vi "AutoAnneal.vi"(0 "VISA resource name":refnum<visa-resource-name>, 1 "Preheat Current":dbl format="%.3f", 5 "Ouput(On:T)":bool=TRUE, 7 "Current Mode(Immediate:F)":bool, 9 "Voltage Mode(Immediate:F)":bool, 11 "error in (no error)":errorcluster, 12 "Voltage":dbl=8.19 format="%.3f", 13 "Preheat Ramp Delay":u32=1000, 14 "Protection(None:0)":u16(ring) items=["None", "Overcurrent protection", "Overvoltage protection", "Overcurrent and overvoltage protection", "Clear overvoltage condition", "Clear overcurrent protection", "Set time delay"]) -> ()   [LabVIEW 2012]
doc: "The Application Example configures, triggers (after a user defined time delay) and stores the setting to a user defined address."
uses:
  Agilent 66XX Series.lvlib
panel:
  in  "Ramp Down Step Size":dbl=0.005 format="%.3f"
  in  "Ramp Down Delay":u32=2000
  in  "Anneal Time":dbl=5.0 format="%.3f"
  out "Anneal Current 2":dbl(graph)
  out "error out":errorcluster
  in  "Preheat Time":dbl=5.0 format="%.3f"
  in  "Overvoltage prot value":dbl=5.0 format="%.3f"
  in  "Anneal Current":dbl format="%.3f"
  in  "Anneal Step Size":dbl=0.005 format="%.3f"
  in  "Anneal Ramp Delay":u32=2000
  out "Anneal Current":dbl(graph)
  out "Preheat Current":dbl(graph)
  in  "START":bool
  in  "Preheat Step Size":dbl=0.1 format="%.3f"
  in  "Reset (F:no)":bool
  in  "ID query (T:yes)":bool=TRUE
  # "Power Supply Configurations"
  # "Preheat Settings"
  # "Amps"
  # "min"
  # "ms"
  # "Amps/Step"
  # "ms"
  # "Anneal Settings"
  # "Ramp Down Settings"
  # "Amps/Step"
  # "Yes"
  # "No"
  # "Yes"
  # "No"
  # "Trigger"
  # "Immediate"
  # "Trigger"
  # "Immediate"
  # "On"
  # "Off"
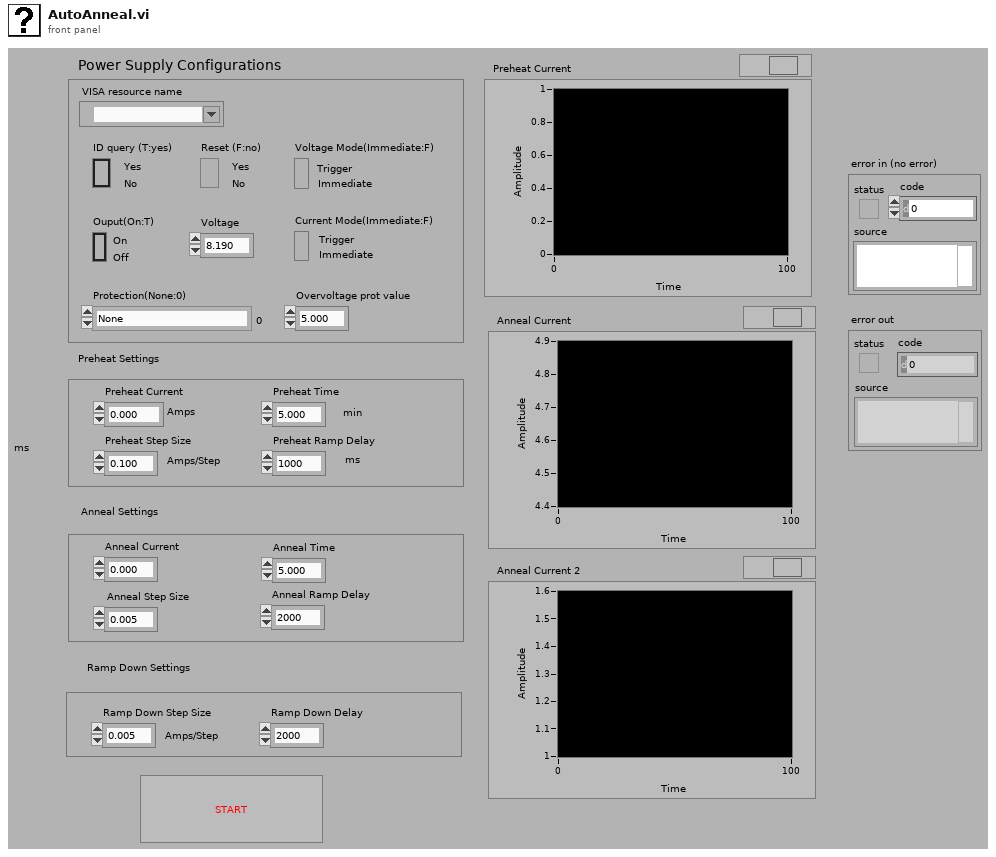
[diagram p1: front panel]
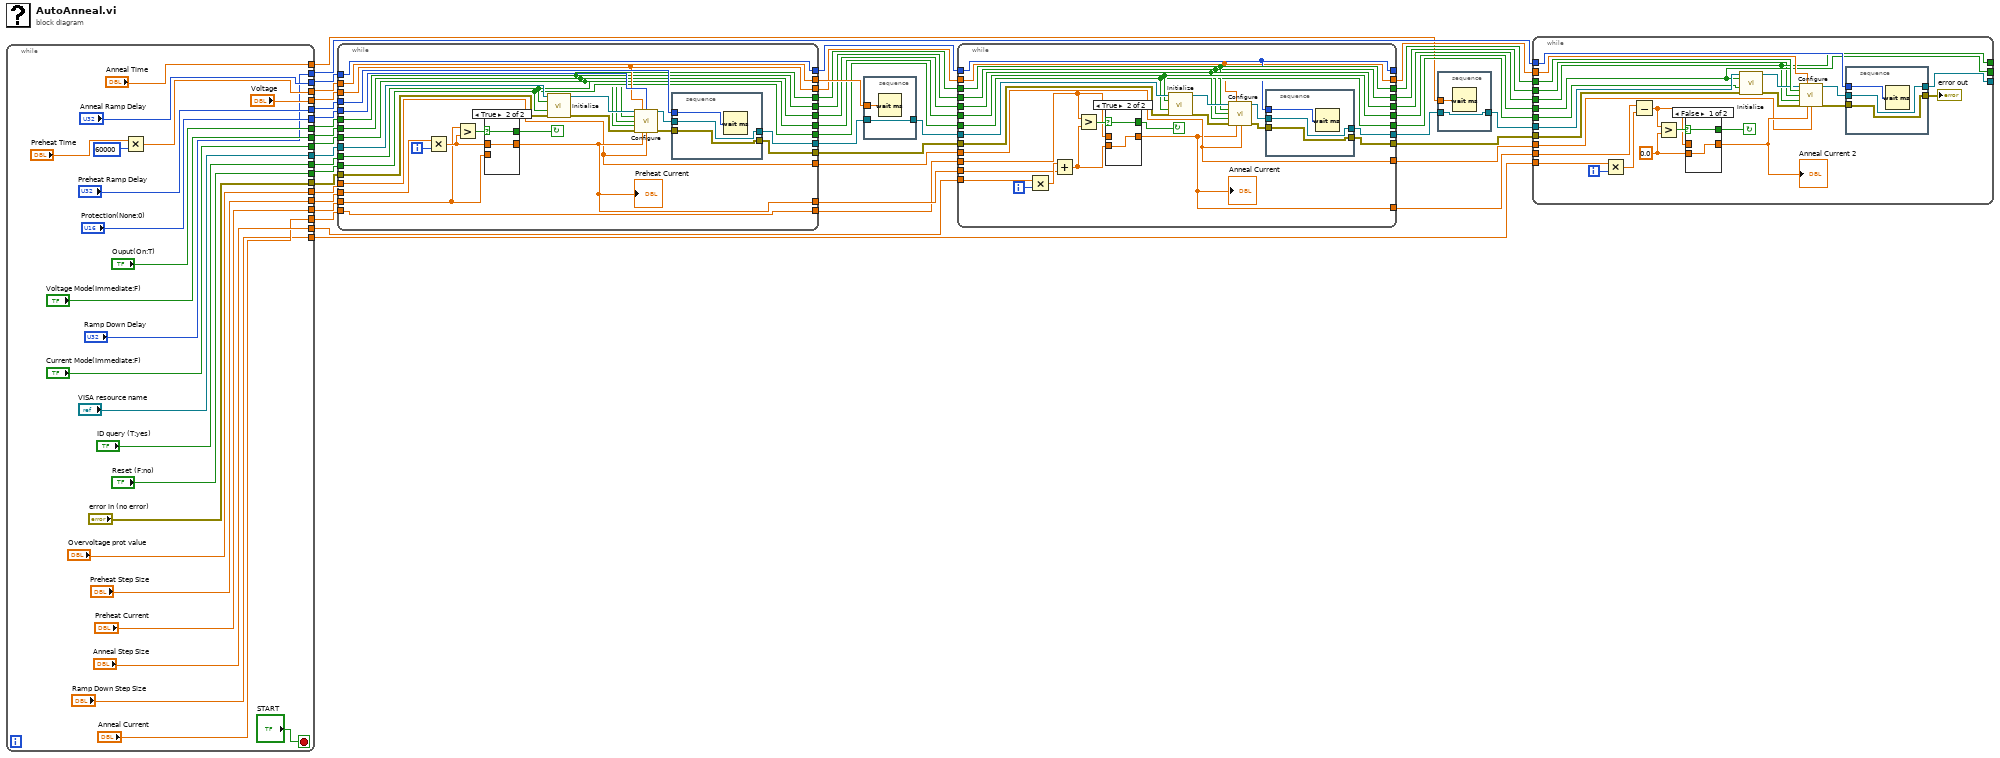
[diagram p0: block diagram]
diagram:
  n1 = while {
    tunnel: ["Current Mode(Immediate:F)"] -> w45
    tunnel: ["Voltage Mode(Immediate:F)"] -> w44
    tunnel: ["Ouput(On:T)"] -> w43
    tunnel: ["Voltage"] -> w42
    tunnel: ["Protection(None:0)"] -> w41
    tunnel: ["Preheat Current"] -> w40
    tunnel: ["Preheat Ramp Delay"] -> w39
    tunnel: ["VISA resource name"] -> w38
    tunnel: ["ID query (T:yes)"] -> w37
    tunnel: ["Reset (F:no)"] -> w36
    tunnel: ["error in (no error)"] -> w35
    tunnel: ["Preheat Step Size"] -> w34
    tunnel: [w50] -> w32
    tunnel: ["Anneal Ramp Delay"] -> w30
    tunnel: ["Anneal Step Size"] -> w24
    tunnel: ["Anneal Current"] -> w22
    tunnel: ["Overvoltage prot value"] -> w16
    tunnel: ["Ramp Down Step Size"] -> w3
    tunnel: ["Ramp Down Delay"] -> w2
    tunnel: ["Anneal Time"] -> w1
    stop <- "START" stop-if-true
    n2 = Multiply(x="Preheat Time", y=60000) -> (x*y=w50:dbl)
  }
  n3 = while {
    tunnel: w45 -> [w73]
    tunnel: w44 -> [w72]
    tunnel: w43 -> [w71]
    tunnel: w42 -> [w80]
    tunnel: w41 -> [w95]
    tunnel: w40 -> [w85]
    tunnel: w39 -> [w93]
    tunnel: w38 -> [w79]
    tunnel: w37 -> [w78]
    tunnel: w36 -> [w77]
    tunnel: w35 -> [w90]
    tunnel: w34 -> [w88]
    tunnel: [w83] -> w33
    tunnel: [w82] -> w31
    tunnel: w32 -> [w82]
    tunnel: w30 -> [w81]
    tunnel: [w81] -> w29
    tunnel: [w80] -> w28
    tunnel: [w78] -> w27
    tunnel: [w77] -> w26
    tunnel: [w76] -> w25
    tunnel: [w75] -> w23
    tunnel: w22 -> [w74]
    tunnel: [w74] -> w21
    tunnel: [w73] -> w19
    tunnel: [w72] -> w18
    tunnel: [w71] -> w17
    tunnel: w16 -> [w69]
    tunnel: [w69] -> w15
    i -> [w89]
    stop <- w84 continue-if-true
    n4 = Multiply(x=w88, y=w89) -> (x*y=w86:dbl)
    n5 = Greater?(x=w85, y=w86) -> (0:w87:bool)
    n6 = case shown="True" w87 {
      selector: w87 -> [w96 w98]
      tunnel: w86 -> [_ w99]
      tunnel: [w97 w99] -> w75
      tunnel: w85 -> [w97 _]
      tunnel: [w96 w98] -> w84
      frame False {
      }
      frame True {
      }
    }
    "Preheat Current" <- w75
    n7 = call "Initialize.vi"("VISA resource name"=w79, "ID query (T:yes)"=w78, "Reset (F:no)"=w77, "error in (no error)"=w90) -> ("VISA resource name out"=w92:refnum<visa-resource-name>, "error out"=w91:errorcluster)  [unwired: 10 in]
    n8 = call "Configure.vi"("VISA resource name"=w92, "Voltage(0 Volts)"=w80, "Protection(None:0)"=w95, "Ouput(On:T)"=w71, "Voltage Mode(F:Immediate)"=w72, "Current Mode(F:Immediate)"=w73, "error in (no error)"=w91, "Current(0 Amps)"=w75, "Overvoltage prot value(50 Volts)"=w69) -> ("VISA resource name out"=w94:refnum<visa-resource-name>, "error out"=w70:errorcluster)  [unwired: 5 in]
    n9 = stacked-sequence {
      tunnel: w94 -> [w102]
      tunnel: w70 -> [w101]
      tunnel: [w102] -> w83
      tunnel: [w101] -> w76
      tunnel: w93 -> [w100]
      frame #0 {
        n10 = Wait (ms)(milliseconds to wait=w100) -> ()  [unwired: 1 out]
      }
    }
  }
  n11 = stacked-sequence {
    tunnel: w33 -> [w104]
    tunnel: [w104] -> w20
    tunnel: w31 -> [w103]
    frame #0 {
      n12 = Wait (ms)(milliseconds to wait=w103) -> ()  [unwired: 1 out]
    }
  }
  n13 = while {
    tunnel: [w114] -> w13
    tunnel: w18 -> [w112]
    tunnel: w17 -> [w113]
    tunnel: w28 -> [w105]
    tunnel: w21 -> [w122]
    tunnel: w29 -> [w108]
    tunnel: w20 -> [w125]
    tunnel: [w119] -> w12
    tunnel: w26 -> [w111]
    tunnel: w24 -> [w107]
    tunnel: [w120] -> w9
    tunnel: w27 -> [w119]
    tunnel: w25 -> [w118]
    tunnel: w23 -> [w116]
    tunnel: w19 -> [w114]
    tunnel: w15 -> [w109]
    tunnel: [w113] -> w11
    tunnel: [w112] -> w10
    tunnel: [w111] -> w8
    tunnel: [w110] -> w7
    tunnel: [w109] -> w6
    tunnel: [w108] -> _
    tunnel: [w106] -> w5
    tunnel: [w105] -> w4
    i -> [w124]
    stop <- w121 continue-if-true
    n14 = Multiply(x=w107, y=w124) -> (x*y=w117:dbl)
    n15 = Add(x=w117, y=w116) -> (x+y=w115:dbl)
    n16 = Greater?(x=w122, y=w115) -> (0:w123:bool)
    n17 = case shown="True" w123 {
      selector: w123 -> [w130 w132]
      tunnel: w115 -> [_ w133]
      tunnel: [w131 w133] -> w106
      tunnel: w122 -> [w131 _]
      tunnel: [w130 w132] -> w121
      frame False {
      }
      frame True {
      }
    }
    "Anneal Current" <- w106
    n18 = call "Initialize.vi"("VISA resource name"=w125, "ID query (T:yes)"=w119, "Reset (F:no)"=w111, "error in (no error)"=w118) -> ("VISA resource name out"=w127:refnum<visa-resource-name>, "error out"=w126:errorcluster)  [unwired: 10 in]
    n19 = call "Configure.vi"("VISA resource name"=w127, "Voltage(0 Volts)"=w105, "Ouput(On:T)"=w113, "Voltage Mode(F:Immediate)"=w112, "Current Mode(F:Immediate)"=w114, "error in (no error)"=w126, "Current(0 Amps)"=w106, "Overvoltage prot value(50 Volts)"=w109) -> ("VISA resource name out"=w129:refnum<visa-resource-name>, "error out"=w128:errorcluster)  [unwired: 6 in]
    n20 = stacked-sequence {
      tunnel: w129 -> [w136]
      tunnel: w128 -> [w135]
      tunnel: [w136] -> w120
      tunnel: [w135] -> w110
      tunnel: w108 -> [w134]
      frame #0 {
        n21 = Wait (ms)(milliseconds to wait=w134) -> ()  [unwired: 1 out]
      }
    }
  }
  n22 = stacked-sequence {
    tunnel: w9 -> [w138]
    tunnel: [w138] -> w14
    tunnel: w1 -> [w137]
    frame #0 {
      n23 = Wait (ms)(milliseconds to wait=w137) -> ()  [unwired: 1 out]
    }
  }
  n24 = while {
    tunnel: [w146] -> _
    tunnel: w11 -> [w163]
    tunnel: w4 -> [w162]
    tunnel: w2 -> [w159]
    tunnel: w14 -> [w156]
    tunnel: [w148] -> _
    tunnel: w8 -> [w155]
    tunnel: w3 -> [w153]
    tunnel: [w149] -> _
    tunnel: w12 -> [w148]
    tunnel: w7 -> [w147]
    tunnel: w13 -> [w146]
    tunnel: w6 -> [w144]
    tunnel: w10 -> [w143]
    tunnel: w5 -> [w141]
    i -> [w154]
    stop <- w151 continue-if-true
    w139 = 0.0
    n25 = Multiply(x=w153, y=w154) -> (x*y=w142:dbl)
    n26 = Subtract(x=w141, y=w142) -> (x-y=w140:dbl)
    n27 = Greater?(x=w140, y=w139) -> (0:w152:bool)
    n28 = case shown="False" w152 {
      selector: w152 -> [w164 w166]
      tunnel: w140 -> [_ w167]
      tunnel: [w165 w167] -> w150
      tunnel: w139 -> [w165 _]
      tunnel: [w164 w166] -> w151
      frame False {
      }
      frame True {
      }
    }
    "Anneal Current 2" <- w150
    n29 = call "Initialize.vi"("VISA resource name"=w156, "ID query (T:yes)"=w148, "Reset (F:no)"=w155, "error in (no error)"=w147) -> ("VISA resource name out"=w158:refnum<visa-resource-name>, "error out"=w157:errorcluster)  [unwired: 10 in]
    n30 = call "Configure.vi"("VISA resource name"=w158, "Voltage(0 Volts)"=w162, "Ouput(On:T)"=w163, "Voltage Mode(F:Immediate)"=w143, "Current Mode(F:Immediate)"=w146, "error in (no error)"=w157, "Current(0 Amps)"=w150, "Overvoltage prot value(50 Volts)"=w144) -> ("VISA resource name out"=w161:refnum<visa-resource-name>, "error out"=w160:errorcluster)  [unwired: 6 in]
    n31 = stacked-sequence {
      tunnel: w161 -> [w170]
      tunnel: w160 -> [w169]
      tunnel: [w170] -> w149
      tunnel: [w169] -> w145
      tunnel: w159 -> [w168]
      frame #0 {
        n32 = Wait (ms)(milliseconds to wait=w168) -> ()  [unwired: 1 out]
      }
    }
    "error out" <- w145
  }
